vi "MESLog_Item_Result.vi"(0 "ItemResultID":string, 1 "ResultID":string, 2 "Barcode":string, 3 "ItemName":string, 4 "ItemIndex":string, 5 "ItemResult":string, 6 "BeginDate":string, 7 "CreateDate":string, 8 "LoopNum":string, 10 "IsChecked":string) -> (16 "Item_Result":string)   [LabVIEW 2014]
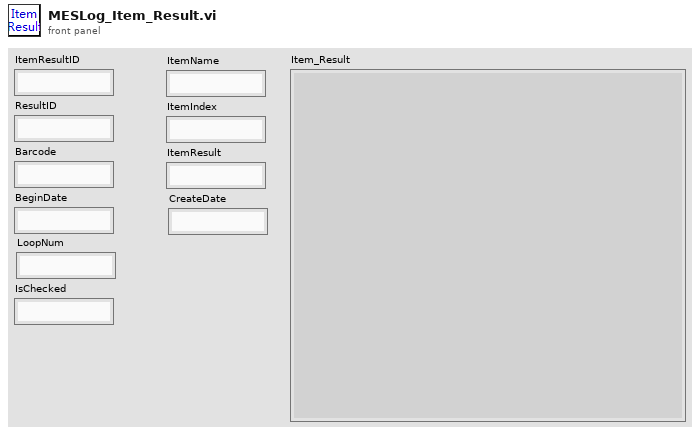
[diagram p1: front panel]
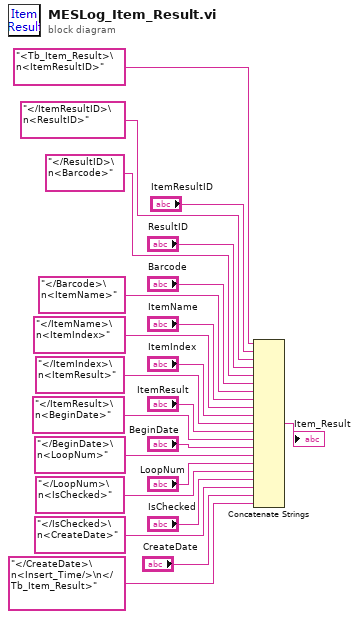
[diagram p0: block diagram]
diagram:
  n1 = Concatenate Strings("<Tb_Item_Result>\n<ItemResultID>" ("string"), "ItemResultID", "</ItemResultID>\n<ResultID>" ("string"), "ResultID", "</ResultID>\n<Barcode>" ("string"), "Barcode", "</Barcode>\n<ItemName>" ("string"), "ItemName", "</ItemName>\n<ItemIndex>" ("string"), "ItemIndex", "</ItemIndex>\n<ItemResult>" ("string"), "ItemResult", "</ItemResult>\n<BeginDate>" ("string"), "BeginDate", "</BeginDate>\n<LoopNum>" ("string"), "LoopNum", "</LoopNum>\n<IsChecked>" ("string"), "IsChecked", "</IsChecked>\n<CreateDate>" ("string"), "CreateDate", "</CreateDate>\n<Insert_Time/>\n</Tb_Item_Result>" ("string")) -> (→"Item_Result":string)
